vi "MongoDB.FindOne.vi"(8 "error in (no error)":errorcluster, 11 "MongoDB.Collection in":refnum<class "MongoDB.Collection.lvclass">) -> (0 "error out":errorcluster, 2 "Result":string, 3 "MongoDB.Collection out":refnum<class "MongoDB.Collection.lvclass">)   [LabVIEW 2014, in "MongoDB.Collection.lvclass"]
uses:
  MongoDB.Collection.lvclass
  MongoDB.Collection.lvclass/MongoDB.Collection.ctl
  C:/Users/Richard/Documents/GitHub/mongo-labview-driver/CSharp/bin/MongoDB.Driver.Legacy.dll
  CSharp/bin/MongoDB.Driver.Legacy.dll
  C:/Users/Richard/Documents/GitHub/mongo-labview-driver/CSharp/bin/MongoDB.Bson.dll
  CSharp/bin/MongoDB.Bson.dll
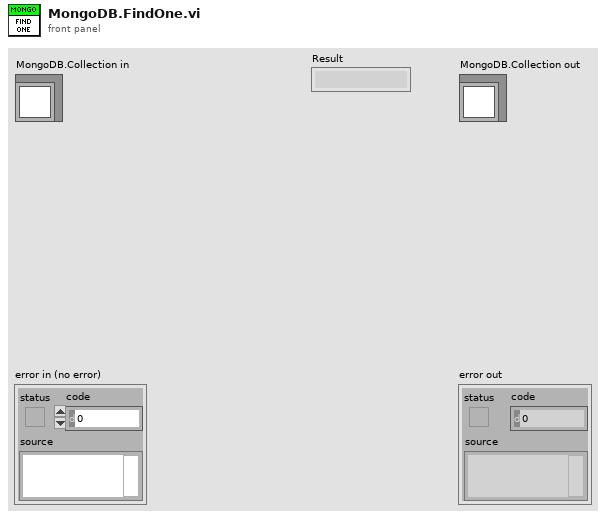
[diagram p1: front panel]
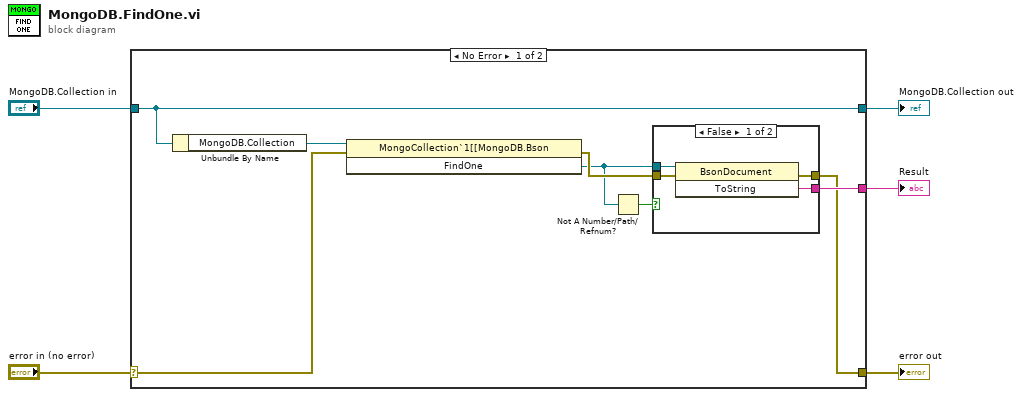
[diagram p0: block diagram]
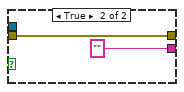
[diagram p2: hidden frame]
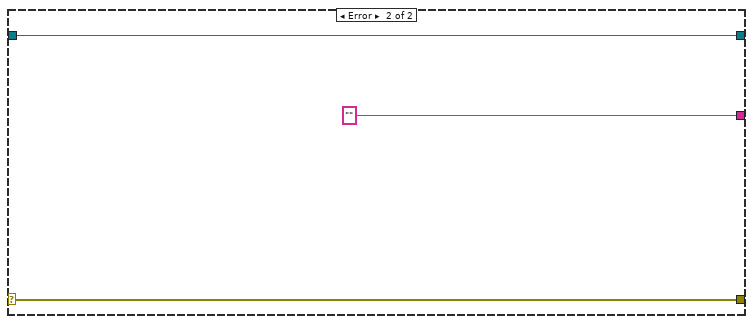
[diagram p3: hidden frame]
diagram:
  n1 = case shown="No Error" "error in (no error)" {
    selector: "error in (no error)" -> [w9 w22]
    tunnel: [w8 w22] -> w4
    tunnel: [w13 w21] -> w2
    tunnel: "MongoDB.Collection in" -> [w13 w21]
    tunnel: [w11 "" ("AsString")] -> w1
    frame No Error {
      n2 = Unbundle By Name(w13) -> ("MongoDB.Collection"=w12:refnum<k24>)
      n3 = invoke class="MongoCollection`1[[MongoDB.Bson" method="FindOne"(reference=w12, error in=w9) -> (error out=w10:errorcluster, "FindOne"=w7:refnum<k24>)  [unwired: 1 in, 1 out]
      n4 = Not A Number/Path/Refnum?(number/path/refnum=w7) -> (NaN/Path/Refnum?=w6:bool)
      n5 = case shown="False" w6 {
        tunnel: [w14 "" ("AsString")] -> w11
        tunnel: w7 -> [w17 _]
        tunnel: w10 -> [w16 w18]
        tunnel: [w15 w18] -> w8
        frame False {
          n6 = invoke class="BsonDocument" method="ToString"(reference=w17, error in=w16) -> (error out=w15:errorcluster, "ToString"=w14:string)  [unwired: 1 in, 1 out]
        }
        frame True {
        }
      }
    }
    frame Error {
    }
  }
  "error out" <- w4
  "MongoDB.Collection out" <- w2
  "Result" <- w1
